vi "Write Data.vi"(6 "Local Data":T1, 8 "error in":errorcluster, 11 "Current Value Table":map{string, dbl}(c390)) -> (0 "error out":errorcluster, 4 "Local Data Out":T1)   [LabVIEW 2025]
uses:
  Controls/Local Data_Recording.ctl
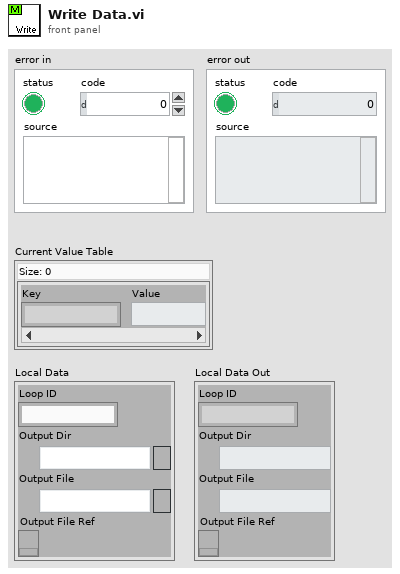
[diagram p1: front panel]
types:
  T1 = typedef "Local Data_Recording.ctl" = cluster{"Loop ID":string, "Output Dir":path, "Output File":path, "Output File Ref":refnum<k34>}
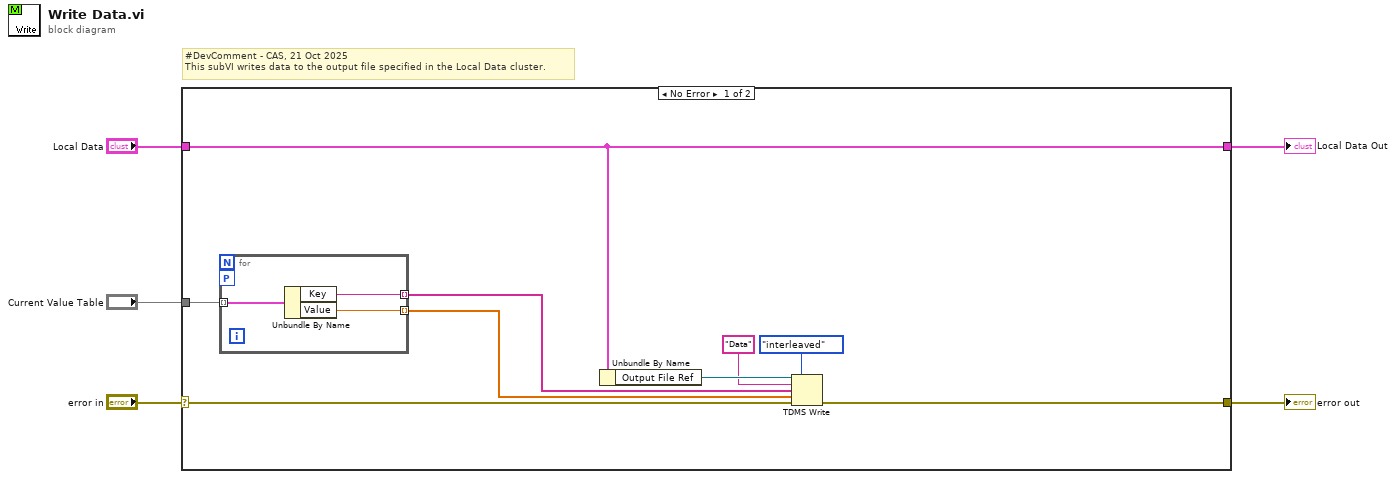
[diagram p0: block diagram]
diagram:
  # "#DevComment - CAS, 21 Oct 2025\nThis subVI writes data to the output file specified in the Local Data cluster."
  n1 = case shown="No Error" "error in" {
    selector: "error in" -> [w13 w19]
    tunnel: [w12 w19] -> w4
    tunnel: [w11 w18] -> w3
    tunnel: "Local Data" -> [w11 w18]
    tunnel: "Current Value Table" -> [w14 _]
    frame No Error {
      n2 = for {
        tunnel: w14 -> [w17] mode=indexing
        workers-P: _ -> [_]
        tunnel: [w16] -> w8 mode=indexing
        tunnel: [w15] -> w7 mode=indexing
        n3 = Unbundle By Name(w17) -> ("Key"=w16:string, "Value"=w15:dbl)
      }
      n4 = Unbundle By Name(w11) -> ("Output File Ref"=w10:refnum<k34>)
      n5 = TDMS Write(0:w10, 1:enum16{"decimated", "interleaved"}."interleaved" ("data layout (0:decimated)"), 5:"Data" ("group name in (Untitled)"), 7:w8, 9:w7, 11:w13) -> (15:w12:errorcluster)  [unwired: 3 out]
    }
    frame Error {
    }
  }
  "error out" <- w4
  "Local Data Out" <- w3
